vi "Exit.vi"(8 "error in (no error)":errorcluster caption="错误输入（无错误）", 11 "VI引用":refnum<vi>) -> (0 "error out":errorcluster caption="错误输出")   [LabVIEW 2011]
panel:
  # "在RunTime时，退出应用程序；在开发模式，关闭vi前面板"
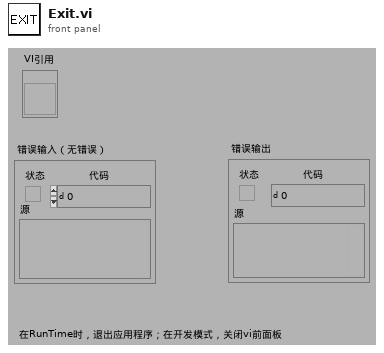
[diagram p1: front panel]
types:
  T1 = enum32{"invalid app kind", "Development System", "Run Time System", "Student Edition", "Embedded LabVIEW", "Evaluation", "Custom"}
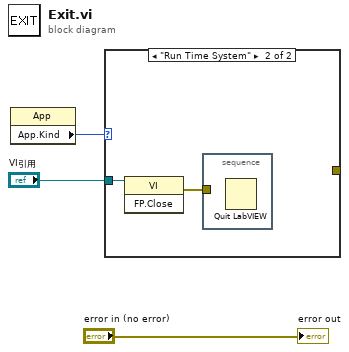
[diagram p0: block diagram]
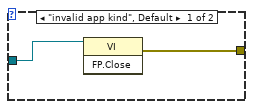
[diagram p2: hidden frame]
diagram:
  n1 = property class="App"() -> ("App.Kind"=w2:T1)  [unwired: 2 in, 2 out]
  n2 = case shown="\"Run Time System\"" w2 {
    tunnel: "VI引用" -> [w5 w7]
    tunnel: [w4 _] -> _
    frame "invalid app kind", Default {
      n3 = invoke class="VI" method="FP.Close"(reference=w5) -> (error out=w4:errorcluster)  [unwired: 2 in, 2 out]
    }
    frame "Run Time System" {
      n4 = invoke class="VI" method="FP.Close"(reference=w7) -> (error out=w6:errorcluster)  [unwired: 2 in, 2 out]
      n5 = stacked-sequence {
        tunnel: w6 -> [_]
        frame #0 {
          n6 = Quit LabVIEW() -> ()  [unwired: 1 in]
        }
      }
    }
  }
  "error out" <- "error in (no error)"
